vi "Read Keys By Name.vi"(8 "error in (no error)":errorcluster, 9 "Search Keys":string[](array[string]), 10 "section":string, 11 "Hardware INI Path":path) -> (0 "error out":errorcluster, 3 "Key Data":string[](array[string]))   [LabVIEW 2017]
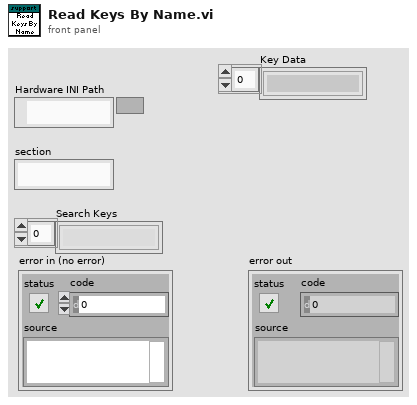
[diagram p1: front panel]
types:
  T1 = enum32{"Read All Sections", "Read Single Section", "Update All Sections", "Create/Update Section"}
  T2 = cluster{"Section Name":string, "Keys":cluster{"Key Name":string, "Key Data":string}[]}[]
  T3 = cluster{"Section Name":string, "Keys":cluster{"Key Name":string, "Key Data":string}[]}
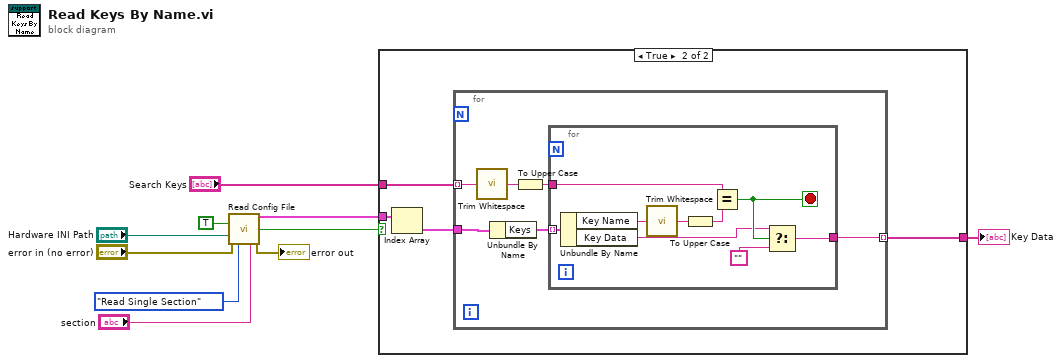
[diagram p0: block diagram]
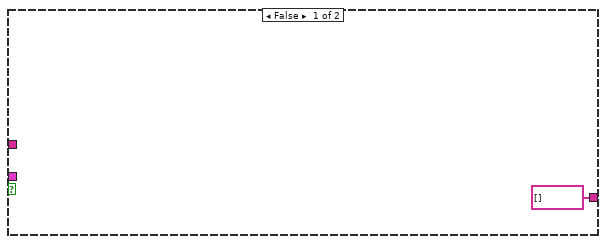
[diagram p2: hidden frame]
diagram:
  n1 = call "Read Config File.vi"("Standalone"=TRUE, "file path (use dialog)"="Hardware INI Path", "error in"="error in (no error)", "All or partial"=T1."Read Single Section", "section (read or create/update)"="section") -> ("INI Data Out"=w7:T2, "found?"=w9:bool, "error out"=→"error out":errorcluster)  [unwired: 4 in, 4 out]
  n2 = case shown="True" w9 {
    tunnel: w7 -> [_ w14]
    tunnel: "Search Keys" -> [_ w13]
    tunnel: [string[] [] w12] -> w3
    frame False {
    }
    frame True {
      n3 = Index Array(array=w14) -> (element=w15:T3)  [unwired: 1 in]
      n4 = for {
        tunnel: w15 -> [w20]
        tunnel: w13 -> [w18] mode=indexing
        tunnel: [w16] -> w12 mode=indexing
        n5 = call <vilib>:"Trim Whitespace.vi"("string"=w18) -> ("trimmed string"=w19:string)  [unwired: 1 in]
        n6 = Unbundle By Name(w20) -> ("Keys"=w21:cluster{"Key Name":string, "Key Data":string}[])
        n7 = To Upper Case(1:w19) -> (0:w17:string)
        n8 = for {
          tunnel: w21 -> [w30] mode=indexing
          tunnel: w17 -> [w27]
          tunnel: [w23] -> w16
          stop <- w25 stop-if-true
          n9 = Unbundle By Name(w30) -> ("Key Name"=w29:string, "Key Data"=w24:string)
          n10 = call <vilib>:"Trim Whitespace.vi"("string"=w29) -> ("trimmed string"=w28:string)  [unwired: 1 in]
          n11 = To Upper Case(1:w28) -> (0:w26:string)
          n12 = Equal?(x=w27, y=w26) -> (x = y?=w25:bool)
          n13 = Select(t=w24, s=w25, f="") -> (s? t:f=w23:string)
        }
      }
    }
  }
  "Key Data" <- w3
